vi "EMC_Retry.vi"(7 "Retry timeout (ms)":i32=10000, 8 "error in (no error)":errorcluster, 10 "Count in":i32) -> (0 "error out":errorcluster, 2 "Exit":bool)   [LabVIEW 2014]
doc: "-77070 Error occured, retry\n(until timeout value reached)"
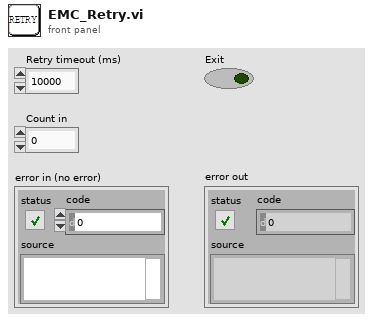
[diagram p1: front panel]
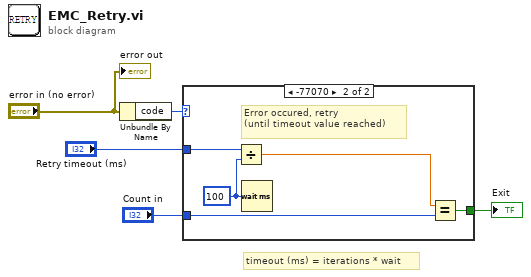
[diagram p0: block diagram]
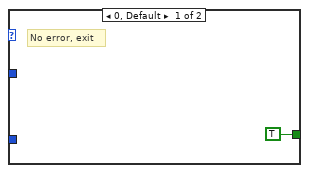
[diagram p2: hidden frame]
diagram:
  # "timeout (ms) = iterations * wait"
  n1 = Unbundle By Name("error in (no error)") -> ("code"=w2:i32)
  n2 = case shown="-77070" w2 {
    tunnel: [TRUE w7] -> w3
    tunnel: "Retry timeout (ms)" -> [_ w10]
    tunnel: "Count in" -> [_ w8]
    frame 0, Default {
      # "No error, exit"
    }
    frame -77070 {
      w11 = u32 100 ("milliseconds to wait")
      # "Error occured, retry\n(until timeout value reached)"
      n3 = Divide(x=w10, y=w11) -> (x/y=w9:dbl)
      n4 = Wait (ms)(milliseconds to wait=w11) -> ()  [unwired: 1 out]
      n5 = Equal?(x=w9, y=w8) -> (x = y?=w7:bool)
    }
  }
  "Exit" <- w3
  "error out" <- "error in (no error)"
